vi "DrawPiePlot.vi"(0 "reference in":refnum<class "HTMLPlot.lvclass">, 1 "PiePlot.PlotLabels":string[](array[string]), 2 "PiePlot.Dataset":dbl[][](array[numeric]), 3 "PiePlot.DatasetLabels":string[](array[string]), 5 "error in (no error)":errorcluster, 6 "GenericPlotOptions":T2, 7 "PiePlot.PlotColours":u32[](array[numeric]), 8 "PiePlotOptions":T1) -> (14 "reference out":refnum<class "HTMLPlot.lvclass">, 19 "error out":errorcluster)   [LabVIEW 2019, in "HTMLPlot.lvclass"]
uses:
  HTMLPlot.lvclass
  Controls/LegendPosition.ctl
  Controls/GenericPlotOptions.ctl
  Controls/PiePlotOptions.ctl
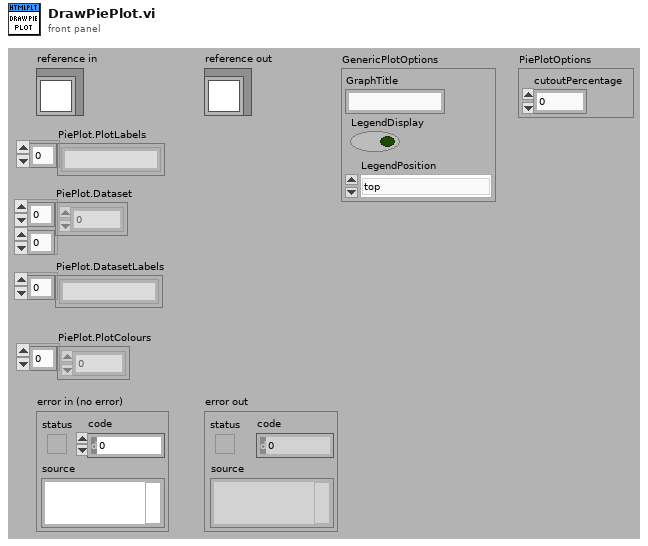
[diagram p1: front panel]
types:
  T1 = typedef "HTMLPlot.lvclass/PiePlotOptions.ctl" = cluster{"cutoutPercentage":i32}
  T2 = typedef "HTMLPlot.lvclass/GenericPlotOptions.ctl" = cluster{"GraphTitle":string, "LegendDisplay":bool, "LegendPosition":T3}
  T3 = typedef "HTMLPlot.lvclass/LegendPosition.ctl" = enum16{"top", "right", "left", "bottom"}
  T4 = cluster{"action":string, "PlotData":string, "GenericPlotOptions":T2, "PiePlotOptions":T1}
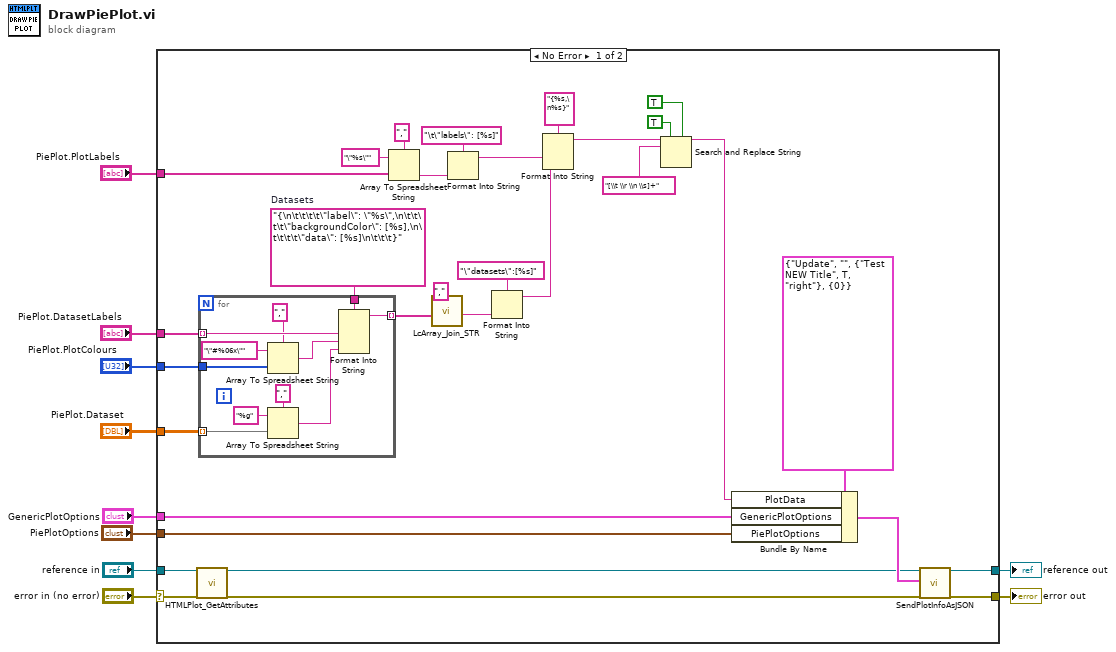
[diagram p0: block diagram]
diagram:
  n1 = case shown="No Error" "error in (no error)" {
    selector: "error in (no error)" -> [w41 w54]
    tunnel: [w12 w54] -> w9
    tunnel: [w14 w53] -> w7
    tunnel: "reference in" -> [w40 w53]
    tunnel: "PiePlot.Dataset" -> [w27 _]
    tunnel: "PiePlot.PlotColours" -> [w26 _]
    tunnel: "PiePlot.DatasetLabels" -> [w25 _]
    tunnel: "PiePlot.PlotLabels" -> [w24 _]
    tunnel: "GenericPlotOptions" -> [w18 _]
    tunnel: "PiePlotOptions" -> [w11 _]
    frame No Error {
      w28 = "{\n\t\t\t\t\"label\": \"%s\",\n\t\t\t\t\"backgroundColor\": [%s],\n\t\t\t\t\"data\": [%s]\n\t\t\t}"  # Datasets
      n2 = call "HTMLPlot_GetAttributes.vi"("reference in"=w40, "error in (no error)"=w41) -> ("reference out"=w15:refnum<class "HTMLPlot.lvclass">, "error out"=w13:errorcluster)  [unwired: 14 in, 2 out]
      n3 = for {
        tunnel: w27 -> [w50] mode=indexing
        tunnel: w26 -> [w43]
        tunnel: w25 -> [w49] mode=indexing
        tunnel: [w47] -> w33 mode=indexing
        tunnel: w28 -> [w46]
        n4 = Array To Spreadsheet String(delimiter (Tab)=",", array=w43, 3:"\"#%06x\"" ("format string")) -> (spreadsheet string=w42:string)
        n5 = Array To Spreadsheet String(delimiter (Tab)=",", array=w50, 3:"%g" ("format string")) -> (spreadsheet string=w48:string)
        n6 = Format Into String(format string=w46, w49, w42, w48) -> (resulting string=w47:string)  [unwired: 2 in, 1 out]
      }
      n7 = Array To Spreadsheet String(delimiter (Tab)=",", array=w24, 3:"\"%s\"" ("format string")) -> (spreadsheet string=w35:string)
      n8 = call "LcArray_Join_STR.vi"("separator"=",", "Array"=w33) -> ("joined string"=w32:string)  [unwired: 8 in, 1 out]
      n9 = Format Into String(format string="\t\"labels\": [%s]", w35) -> (resulting string=w38:string)  [unwired: 2 in, 1 out]
      n10 = Format Into String(format string="\"datasets\":[%s]", w32) -> (resulting string=w30:string)  [unwired: 2 in, 1 out]
      n11 = Format Into String(format string="{%s,\n%s}", w38, w30) -> (resulting string=w17:string)  [unwired: 2 in, 1 out]
      n12 = Search and Replace String(replace all?=TRUE ("replace all? (F)"), multiline?=TRUE ("multiline? (F)"), input string=w17, search string="[\\t \\r \\n \\s]+") -> (result string=w23:string)  [unwired: 4 in, 3 out]
      n13 = Bundle By Name(cluster=T4 {"action"="Update", "PlotData"="", "GenericPlotOptions"={"GraphTitle"="Test NEW Title", "LegendDisplay"=TRUE, "LegendPosition"=enum."right"}, "PiePlotOptions"={"cutoutPercentage"=0}}, "PlotData"=w23, "GenericPlotOptions"=w18, "PiePlotOptions"=w11) -> (w16:T4)
      n14 = call "SendPlotInfoAsJSON.vi"("reference in"=w15, "PlotInfo"=w16, "error in (no error)"=w13) -> ("reference out"=w14:refnum<class "HTMLPlot.lvclass">, "error out"=w12:errorcluster)  [unwired: 15 in]
    }
    frame Error {
    }
  }
  "error out" <- w9
  "reference out" <- w7
